vi "Table Parent ID by Child ID.vi"(8 "error in (no error)":errorcluster) -> (0 "error out":errorcluster, 3 "Table Parent ID by Child ID":variant)   [LabVIEW 2023]
doc: "<b> </b> <b> </b>\n© 2017 Q Software Innovations, LLC\nwritten by Quentin \"Q\" Alldredge\nproduced in LabVIEW 2015\n\nsupport@qsoftwareinnovations.com\nwww.qsoftwareinnovations.com\n\nAll rights reserved.\n\nRedistribution and use in source and binary forms, with or without modification, are permitted provided that the following conditions are met:\n\n * Redistributions of source code must retain the above copyright notice, this list of conditions and the following disclaimer.\n * Redistributions in binary form must reproduce the above copyright notice, this list of conditions and the following disclaimer in the documentation and/or other materials provided with the distribution.\n * Neither the name of Q Software Innovations, LLC. nor the names of its contributors may be used to endorse or promote products derived from this software without specific prior written permission.\n\nTHIS SOFTWARE IS PROVIDED BY THE COPYRIGHT HOLDERS AND CONTRIBUTORS \"AS IS\" AND ANY EXPRESS OR IMPLIED WARRANTIES, INCLUDING, BUT NOT LIMITED TO, THE IMPLIED WARRANTIES OF MERCHANTABILITY AND FITNESS FOR A PARTICULAR PURPOSE ARE DISCLAIMED. IN NO EVENT SHALL THE COPYRIGHT OWNER OR CONTRIBUTORS BE LIABLE FOR ANY DIRECT, INDIRECT, INCIDENTAL, SPECIAL, EXEMPLARY, OR CONSEQUENTIAL DAMAGES (INCLUDING, BUT NOT LIMITED TO, PROCUREMENT OF SUBSTITUTE GOODS OR SERVICES; LOSS OF USE, DATA, OR PROFITS; OR BUSINESS INTERRUPTION) HOWEVER CAUSED AND ON ANY THEORY OF LIABILITY, WHETHER IN CONTRACT, STRICT LIABILITY, OR TORT (INCLUDING NEGLIGENCE OR OTHERWISE) ARISING IN ANY WAY OUT OF THE USE OF THIS SOFTWARE, EVEN IF ADVISED OF THE POSSIBILITY OF SUCH DAMAGE."
panel:
  out "exe time (ms)":u32
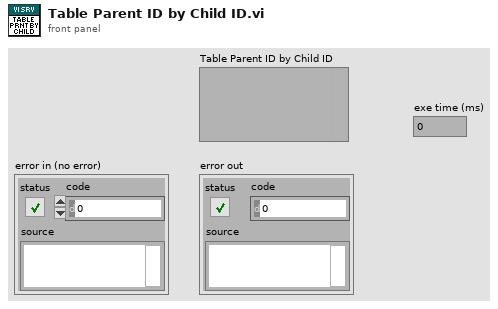
[diagram p1: front panel]
types:
  T1 = cluster{"Unique ID string":string, "Parent ID string":string, "Class Name (unlocalized)":string, "Class Name (localized)":string}[]
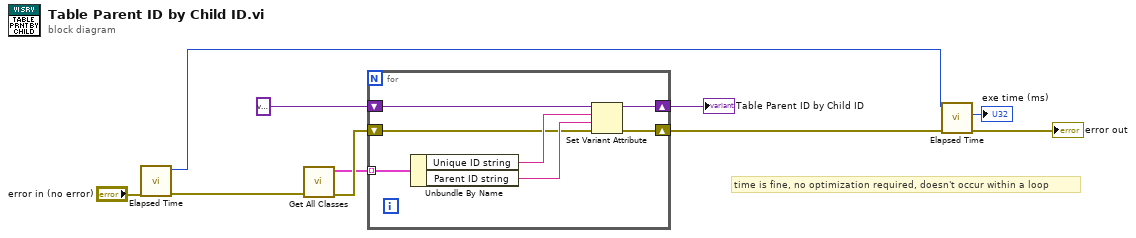
[diagram p0: block diagram]
diagram:
  # "time is fine, no optimization required, doesn't occur within a loop"
  n1 = call "Elapsed Time.vi"("error in"="error in (no error)") -> ("error out"=w5:errorcluster, "millisecond timer value"=w2:u32)  [unwired: 7 in, 2 out]
  n2 = call "Get All Classes.vi"("error in (no error)"=w5) -> ("error out"=w9:errorcluster, "VI Server Classes[]"=w7:T1)  [unwired: 9 in]
  n3 = for {
    tunnel: w7 -> [w17] mode=indexing
    shift-right: [w13] -> w10
    shift-left: variant -> [w16]
    shift-right: [w12] -> w4
    shift-left: w9 -> [w11]
    n4 = Unbundle By Name(w17) -> ("Unique ID string"=w15:string, "Parent ID string"=w14:string)
    n5 = Set Variant Attribute(Variant=w16, name=w15, value=w14, error in=w11) -> (Variant out=w13:variant, error out=w12:errorcluster)  [unwired: 1 out]
  }
  "Table Parent ID by Child ID" <- w10
  n6 = call "Elapsed Time.vi"("error in"=w4, "past time"=w2) -> ("error out"=→"error out":errorcluster, "elapsed time (ms)"=→"exe time (ms)":u32)  [unwired: 6 in, 2 out]
